vi "Write Log (Parent).vi"(5 "Options":T1={"timestamp (now)"=0.0, "Call chain (here)"="", "Count (1)"=1, "Font (override)"={"Font Name"="", "Size"=0, "Bold"=FALSE, "Italic"=FALSE, "Underline"=FALSE, "Strikeout"=FALSE, "Color"=0}, "Add row separator? (T)"=TRUE}, 7 "Logging level (INFO)":T3=enum."INFO", 8 "error in (no error)":errorcluster, 9 "Message":variant, 10 "Message Title":string, 11 "BlueLogParent in":refnum<class "BlueLogParent_OpenSource.lvclass">) -> (0 "error out":errorcluster, 3 "BlueLogParent out":refnum<class "BlueLogParent_OpenSource.lvclass">)   [LabVIEW 2020, in "BlueLogParent_OpenSource.lvclass"]
uses:
  BlueLogParent_OpenSource.lvclass
  BlueLogParentLevel.ctl
  BlueLogParentOptions.ctl
  BlueLogParentFont.ctl
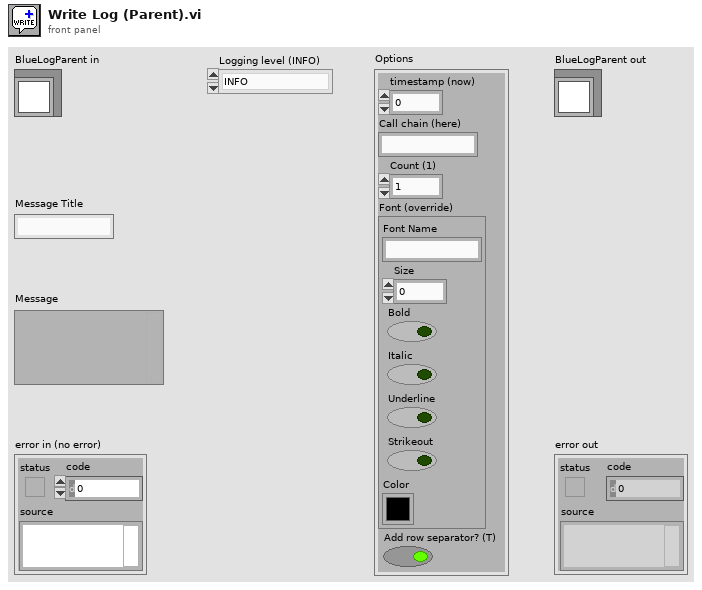
[diagram p1: front panel]
types:
  T1 = typedef "BlueLogParent_OpenSource.lvclass/BlueLogParentOptions.ctl" = cluster{"timestamp (now)":dbl, "Call chain (here)":string, "Count (1)":u16, "Font (override)":T2, "Add row separator? (T)":bool}
  T2 = typedef "BlueLogParent_OpenSource.lvclass/BlueLogParentFont.ctl" = cluster{"Font Name":string, "Size":u16, "Bold":bool, "Italic":bool, "Underline":bool, "Strikeout":bool, "Color":u32}
  T3 = typedef "BlueLogParent_OpenSource.lvclass/BlueLogParentLevel.ctl" = enum16{"DEBUG", "INFO", "WARNING", "ERROR", "CRITICAL"}
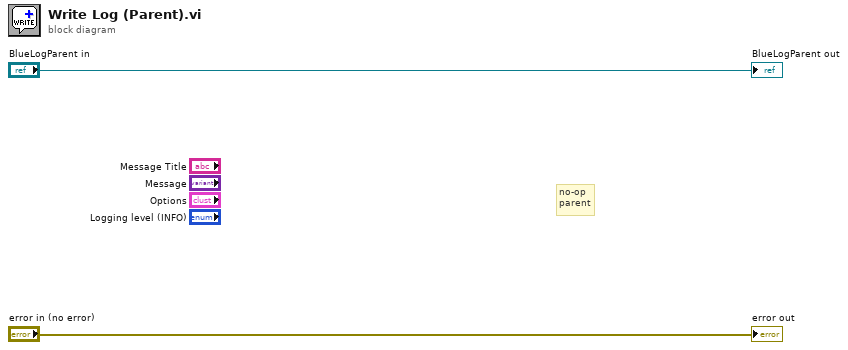
[diagram p0: block diagram]
diagram:
  # "no-op\nparent"
  "error out" <- "error in (no error)"
  "BlueLogParent out" <- "BlueLogParent in"
